vi "kinect_mode.vi"(4 "right left/right":refnum<vi>, 5 "left up/down":refnum<vi>, 6 "right up/down":refnum<vi>, 7 "left left/right":refnum<vi>, 8 "spine Z":refnum<vi>, 9 "Spine X":refnum<vi>) -> (0 "OutputZ":dbl, 1 "OutputX":dbl, 2 "Command":string, 3 "Speed":u8, 11 "Power":bool)   [LabVIEW 2014]
panel:
  out "Getting base position":bool
  out "XY Graph":cluster{"Y":dbl[], "Y":dbl[]}[](graph)
  out "baseX":dbl
  out "baseZ":dbl
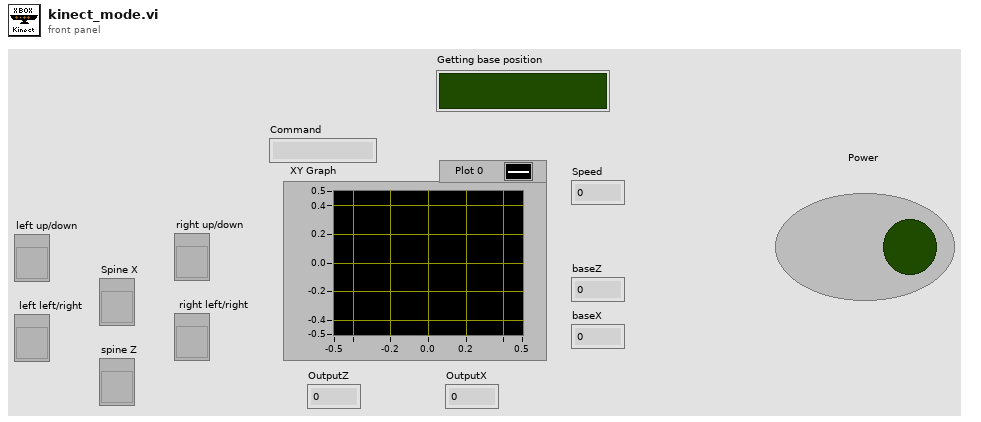
[diagram p1: front panel]
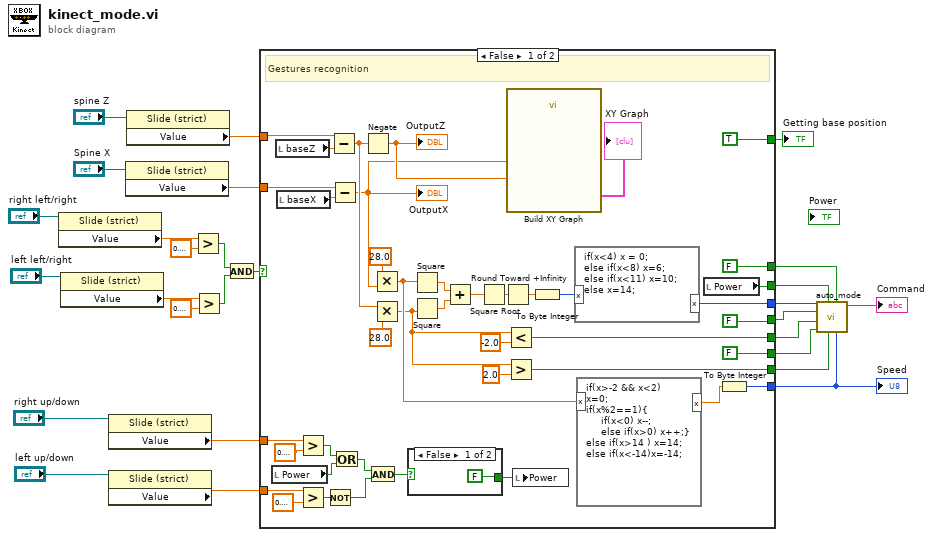
[diagram p0: block diagram]
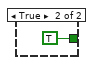
[diagram p2: hidden frame]
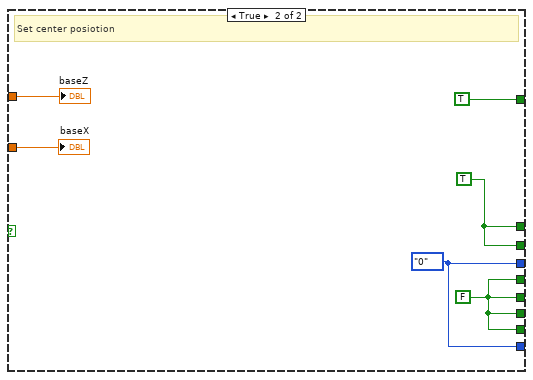
[diagram p3: hidden frame]
diagram:
  n1 = property class="Slide (strict)"(reference="right left/right") -> ("Value"=w25:sgl)  [unwired: 1 in, 2 out]
  n2 = property class="Slide (strict)"(reference="left left/right") -> ("Value"=w21:sgl)  [unwired: 1 in, 2 out]
  n3 = property class="Slide (strict)"(reference="right up/down") -> ("Value"=w1:sgl)  [unwired: 1 in, 2 out]
  n4 = property class="Slide (strict)"(reference="left up/down") -> ("Value"=w2:sgl)  [unwired: 1 in, 2 out]
  n5 = property class="Slide (strict)"(reference="Spine X") -> ("Value"=w7:sgl)  [unwired: 1 in, 2 out]
  n6 = property class="Slide (strict)"(reference="spine Z") -> ("Value"=w8:sgl)  [unwired: 1 in, 2 out]
  n7 = Greater?(x=w25, y=sgl 0.4) -> (0:w24:bool)
  n8 = Greater?(x=w21, y=sgl 0.4) -> (0:w20:bool)
  n9 = And(x=w24, y=w20) -> (x .and. y?=w23:bool)
  n10 = case "Set center position" shown="False" w23 {
    tunnel: [w57 w76] -> w17
    tunnel: [FALSE w74] -> w16
    tunnel: [w41 w74] -> w15
    tunnel: [FALSE w74] -> w14
    tunnel: [w40 w74] -> w13
    tunnel: [w47 w76] -> w5
    tunnel: [w28 w75] -> w12
    tunnel: [FALSE w75] -> w11
    tunnel: w8 -> [w63 w73]
    tunnel: w7 -> [w61 w72]
    tunnel: [TRUE ("Getting base position") TRUE ("Getting base position")] -> w6
    tunnel: w2 -> [w37 _]
    tunnel: w1 -> [w39 _]
    frame False {
      # "Gestures recognition"
      n11 = local read "Power"() -> (w34:bool)
      n12 = local read "baseZ"() -> (w64:dbl)
      n13 = local read "baseX"() -> (w62:dbl)
      n14 = Greater?(x=w39, y=sgl 0.4) -> (0:w35:bool)
      n15 = Greater?(x=w37, y=sgl 0.4) -> (0:w32:bool)
      n16 = Not(x=w32) -> (.not. x?=w30:bool)
      n17 = Subtract(x=w63, y=w64) -> (x-y=w51:dbl)
      n18 = Subtract(x=w61, y=w62) -> (x-y=w43:dbl)
      "OutputX" <- w43
      n19 = Or(x=w35, y=w34) -> (x .or. y?=w31:bool)
      n20 = Negate(x=w51) -> (-x=w50:dbl)
      "OutputZ" <- w50
      n21 = And(x=w31, y=w30) -> (x .and. y?=w29:bool)
      n22 = Multiply(x=28.0, y=w43) -> (x*y=w49:dbl)
      n23 = Multiply(x=w51, y=28.0) -> (x*y=w42:dbl)
      n24 = case shown="False" w29 {
        tunnel: [FALSE TRUE] -> w33
        frame False {
        }
        frame True {
        }
      }
      n25 = Square(x=w49) -> (x^2=w56:dbl)
      n26 = Square(x=w42) -> (x^2=w55:dbl)
      n27 = Add(x=w56, y=w55) -> (x+y=w54:dbl)
      n28 = Square Root(x=w54) -> (sqrt(x)=w60:dbl)
      n29 = Round Toward +Infinity(x=w60) -> (ceil(x): smallest int >= x=w58:dbl)
      n30 = Less?(x=w42, y=-2.0) -> (x < y?=w41:bool)
      n31 = Greater?(x=w42, y=2.0) -> (0:w40:bool)
      n32 = call "Build XY Graph"("Y Input"=w50, "X Input"=w43) -> ("XY Graph"=→"XY Graph":cluster{"X":dbl[], "Y":dbl[]}[])  [unwired: 8 in, 1 out]
      n33 = local write "Power"(w33) -> ()
      n34 = To Byte Integer(number=w58) -> (8bit integer=w59:i8)
      n35 = formula code="if(x<4) x = 0;\nelse if(x<8) x=6;\nelse if(x<11) x=10;\nelse x=14;"("x"=w59) -> ("x"=w57:i8)
      n36 = formula code="if(x>-2 && x<2)\nx=0;\nif(x%2==1){\n     if(x<0) x--;\n     else if(x>0) x++;}\nelse if(x>14 ) x=14;\nelse if(x<-14)x=-14;"("x"=w49) -> ("x"=w48:dbl)
      n37 = local read "Power"() -> (w28:bool)
      n38 = To Byte Integer(number=w48) -> (8bit integer=w47:i8)
    }
    frame True {
      w74 = FALSE
      w75 = TRUE
      w76 = enum16{"0"}."0"
      # "Set center posiotion"
      "baseZ" <- w73
      "baseX" <- w72
    }
  }
  "Getting base position" <- w6
  "Speed" <- w5
  n39 = call "auto_mode.vi"("Curve"=w5, "Base Position"=w11, "Back"=w13, "POWER"=w12, "Right"=w14, "Forth"=w15, "Left"=w16, "Speed"=w17) -> ("String"=→"Command":string)  [unwired: 3 in]
